vi "获取实际值.vi"(10 "字符串":string) -> (0 "实际值字符串":string, 3 "实际值":u32)   [LabVIEW 2016]
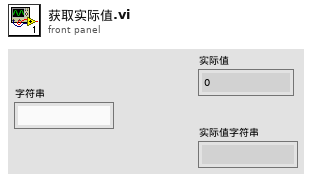
[diagram p1: front panel]
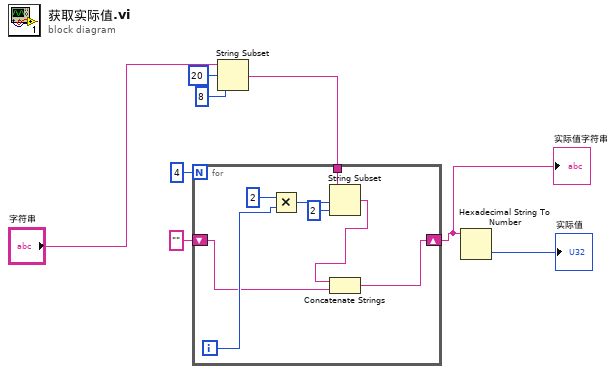
[diagram p0: block diagram]
diagram:
  n1 = String Subset(string="字符串", offset (0)=20 ("偏移量(0)"), length (rest)=8 ("长度（剩余）")) -> (substring=w3:string)
  n2 = for {
    N: 4 -> [_]
    shift-right: [w16] -> w2
    shift-left: "" -> [w9]
    tunnel: w3 -> [w15]
    i -> [w14]
    n3 = Multiply(x=2, y=w14) -> (x*y=w12:i32)
    n4 = String Subset(string=w15, offset (0)=w12, length (rest)=2 ("长度（剩余）")) -> (substring=w10:string)
    n5 = Concatenate Strings(w10, w9) -> (w16:string)
  }
  "实际值字符串" <- w2
  n6 = Hexadecimal String To Number(string=w2) -> (number=→"实际值":u32)  [unwired: 2 in, 1 out]
